vi "VRM_sweepVsg_IV.vi"(7 "Sweep rate (T/min)":dbl=1.0 min=0.0 max=1.0 step=0.01, 8 "Comments":string="SA02703G.20140703\n\nVbg=0V\nsweep Vsg3(cavity): -100mV to 100mV 0.5mV steps\n\nLockin0:18\n1: 19\n2: 21\n3: 22\n4: 23\n5: 24", 9 "Experiment folder name":string="2 - sweep Vsg3", 11 "Parameters":T1={"R1"=0.8, "R2"=0.8, "Theta1 (deg)"=0.0, "Theta2 (deg)"=90.0, "Phi1 (deg)"=90.0, "Phi2 (deg)"=90.0, "Step Size (T/deg/deg)"=15.0, "Stepping Parameter"=enum."Theta"} {"Phi2 (deg)" format="%#_13g"; "Phi1 (deg)" format="%#_13g"; "Theta2 (deg)" format="%#_13g"; "Theta1 (deg)" format="%#_13g"; "R2" format="%#_13g"; "R1" format="%#_13g"}) -> ()   [LabVIEW 2013]
panel:
  in  "Offset":dbl min=-5.0 max=5.0 step=0.01
  in  "Max Field for Triangle":dbl=1.05 min=-2.0 max=2.0 step=0.01
  in  "Ring":u16(ring)=1 items=["Constant Field Sweep", "R - trangle wave"]
  in  "OK Button":bool
  in  "stop":bool
  # "Theta: Azimuthal \nPhi: Polar (from Z down)\nThe ordering is the same as VRM."
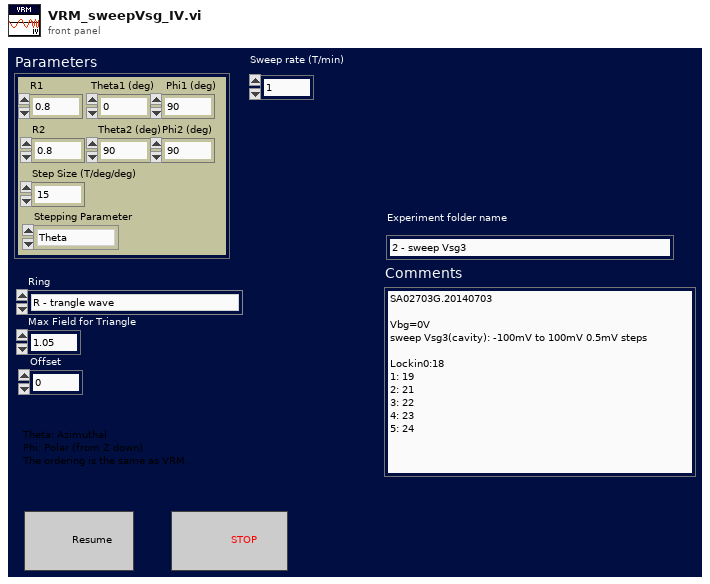
[diagram p1: front panel]
types:
  T1 = cluster{"R1":dbl, "R2":dbl, "Theta1 (deg)":dbl, "Theta2 (deg)":dbl, "Phi1 (deg)":dbl, "Phi2 (deg)":dbl, "Step Size (T/deg/deg)":dbl, "Stepping Parameter":enum16{"R", "Theta", "Phi"}}
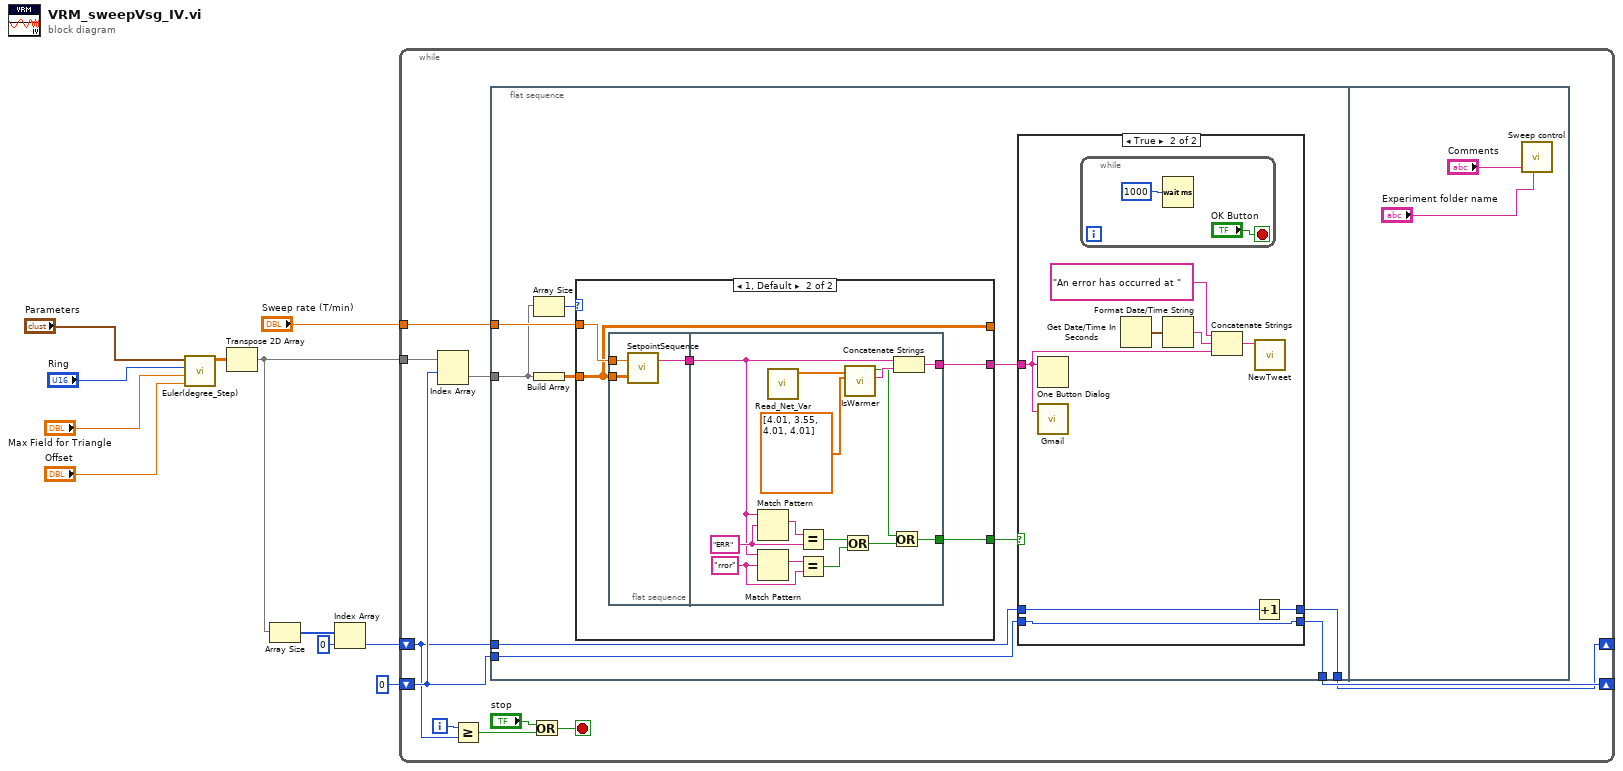
[diagram p0: block diagram]
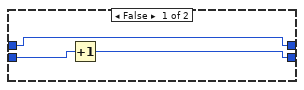
[diagram p2: hidden frame]
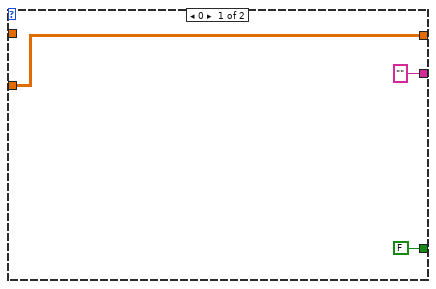
[diagram p3: hidden frame]
diagram:
  n1 = call "Euler(degree_Step).vi"("Offset"="Offset", "Max Field for Triangle"="Max Field for Triangle", "Ring"="Ring", "Cluster"="Parameters") -> ("Waveform Graph"=w9:dbl[][])  [unwired: 7 in]
  n2 = Transpose 2D Array(2D array=w9) -> (transposed array=w5:dbl[][])
  n3 = Array Size(array=w5) -> (size(s)=w7:i32[])
  n4 = Index Array(array=w7, index=0) -> (element=w6:i32)
  n5 = while {
    tunnel: "Sweep rate (T/min)" -> [w22]
    tunnel: w5 -> [w17]
    shift-right: [w14] -> _
    shift-left: 0 -> [w15]
    shift-right: [w12] -> _
    shift-left: w6 -> [w13]
    i -> [w18]
    stop <- w19 stop-if-true
    n6 = Index Array(array=w17, index (row)=w15) -> (element=w16:dbl[])  [unwired: 1 in]
    n7 = Greater Or Equal?(x=w18, y=w13) -> (x >= y?=w21:bool)
    n8 = flat-sequence {
      tunnel: w22 -> [w32]
      tunnel: w16 -> [w31]
      tunnel: w15 -> [w27]
      tunnel: [w26] -> w14
      tunnel: w13 -> [w25]
      tunnel: [w24] -> w12
      frame #0 {
        n9 = Array Size(array=w31) -> (size(s)=w30:i32)
        n10 = Build Array(w31) -> (w29:dbl[][])
        n11 = case shown="1, Default" w30 {
          tunnel: w32 -> [_ w53]
          tunnel: w29 -> [w48 w52]
          tunnel: [w48 w52] -> _
          tunnel: [FALSE w50] -> w28
          tunnel: ["" ("Status") w49] -> w23
          frame 0 {
          }
          frame 1, Default {
            n12 = flat-sequence {
              tunnel: w53 -> [w56]
              tunnel: w52 -> [w55]
              tunnel: [w54] -> w51
              tunnel: w51 -> [w63]
              tunnel: [w58] -> w50
              tunnel: [w61] -> w49
              frame #0 {
                n13 = call "SetpointSequence.vi"("appended array"=w55, "Sweep rate (T/min)"=w56) -> ("Status"=w54:string)  [unwired: 1 in]
              }
              frame #1 {
                w67 = "rror" ("regular expression")
                w69 = "ERR" ("regular expression")
                n14 = Match Pattern(string=w63, regular expression=w69) -> (match substring=w70:string)  [unwired: 1 in, 3 out]
                n15 = Match Pattern(string=w63, regular expression=w67) -> (match substring=w68:string)  [unwired: 1 in, 3 out]
                n16 = call "Read_Net_Var.vi"() -> ("Array"=w57:dbl[])  [unwired: 11 in]
                n17 = Equal?(x=w70, y=w69) -> (x = y?=w66:bool)
                n18 = Equal?(x=w68, y=w67) -> (x = y?=w65:bool)
                n19 = Or(x=w66, y=w65) -> (x .or. y?=w60:bool)
                n20 = call "IsWarmer.vi"("Alert Threshold"=dbl[] [4.01, 3.55, 4.01, 4.01], "Temperature In"=w57) -> ("String"=w62:string, "Temperature is above threshold"=w59:bool)  [unwired: 8 in]
                n21 = Or(x=w59, y=w60) -> (x .or. y?=w58:bool)
                n22 = Concatenate Strings(w63, w62) -> (w61:string)
              }
            }
          }
        }
        n23 = case shown="True" w28 {
          tunnel: w27 -> [w35 w43]
          tunnel: [w34 w43] -> w26
          tunnel: w25 -> [w33 w42]
          tunnel: [w33 w41] -> w24
          tunnel: w23 -> [_ w36]
          frame False {
            n24 = Increment(x=w35) -> (x+1=w34:i32)
          }
          frame True {
            n25 = One Button Dialog(message=w36) -> ()  [unwired: 1 in, 1 out]
            n26 = call "Gmail.vi"("Message Main Body"=w36) -> ()  [unwired: 3 in]
            n27 = while {
              stop <- "OK Button" stop-if-true
              n28 = Wait (ms)(milliseconds to wait=u32 1000) -> ()  [unwired: 1 out]
            }
            n29 = Get Date/Time In Seconds() -> (seconds since 1Jan1904=w40:timestamp)
            n30 = Format Date/Time String(seconds (now)=w40) -> (date/time string=w39:string)  [unwired: 2 in]
            n31 = Concatenate Strings("An error has occurred at " ("string"), w39, w36) -> (w38:string)
            n32 = Increment(x=w42) -> (x+1=w41:i32)
            n33 = call "NewTweet.vi"("Message Main Body"=w38) -> ()  [unwired: 11 in]
          }
        }
      }
      frame #1 {
        n34 = call <userlib>:"Sweep control.vi"("Comments"="Comments", "Experiment folder name"="Experiment folder name") -> ()  [unwired: 7 in]
      }
    }
    n35 = Or(x="stop", y=w21) -> (x .or. y?=w19:bool)
  }
